vi "Read ICDAS2ModelColumns.vi"(8 "error in (no error)":errorcluster, 11 "AcPwrSimBase in":refnum<class "AcPwrSimBase.lvclass">) -> (0 "error out":errorcluster, 2 "ICDAS2ModelColumns":string[](array[string]), 3 "AcPwrSimBase out":refnum<class "AcPwrSimBase.lvclass">)   [LabVIEW 2018, in "AcPwrPlugins.lvlib" / "AcPwrSimBase.lvclass"]
uses:
  AcPwrSimBase.lvclass
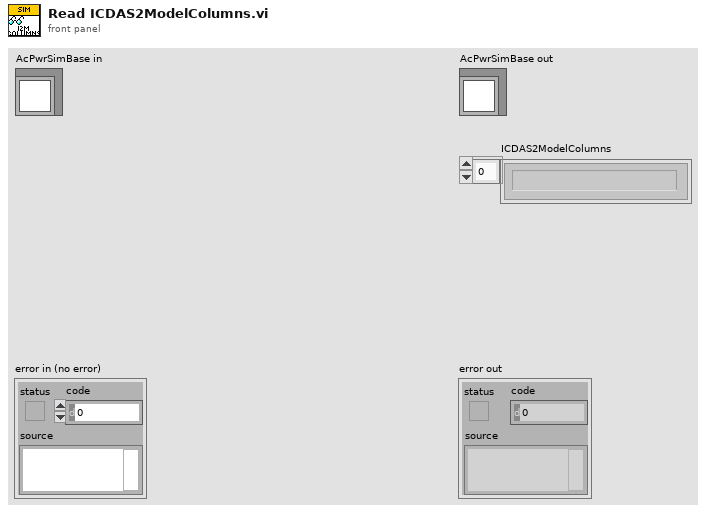
[diagram p1: front panel]
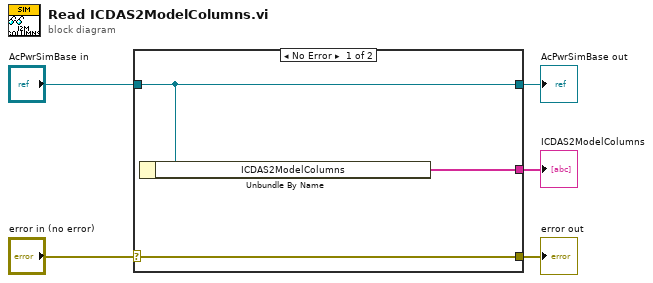
[diagram p0: block diagram]
diagram:
  n1 = case shown="No Error" "error in (no error)" {
    selector: "error in (no error)" -> [w8 w9]
    tunnel: [w8 w9] -> w4
    tunnel: [w7 w10] -> w2
    tunnel: "AcPwrSimBase in" -> [w7 w10]
    tunnel: [w6 _] -> w1
    frame No Error {
      n2 = Unbundle By Name(w7) -> ("ICDAS2ModelColumns"=w6:string[])
    }
    frame Error {
    }
  }
  "error out" <- w4
  "AcPwrSimBase out" <- w2
  "ICDAS2ModelColumns" <- w1
